vi "Car Wash Client.vi"() -> ()   [LabVIEW 2024]
uses:
  Control 1.ctl
  Global Varibles.vi
  <vilib>/Utility/file.llb/Write Delimited Spreadsheet (string).vi
panel:
  out "error out":errorcluster
  in  "Main Tab":T1(tab)
  in  "Register Button":bool
  in  "Login Button":bool
  in  "Login Back Button":bool
  in  "Login Password":string
  in  "Login Username":string
  out "Login LED":bool
  in  "Login User Button":bool
  in  "Register Username":string
  in  "Register Password":string
  in  "Register Back Button":bool
  in  "Register User Button":bool
  in  "Economy Wash Button":bool
  in  "Deluxe Wash Button":bool
  out "Elapsed Time":dbl
  out "Car Wash Main Tab":enum32{"Deluxe 1"}(tab)
  in  "Stop Button":bool
  out "Vehicle Out of Position":bool
  in  "Car Wash Indicators":enum32{"Page 1"}(tab)
  out "Under Body Wash":bool
  out "Soap Application":bool
  out "Main High Pressure Wash":bool
  out "Clear Water Rinse":bool
  out "Air Dry":bool
  out "Car Wash Simulation Switches":enum32{"Page 1", "Page 2"}(tab)
  in  "Air Dry Position Switch":bool
  in  "Main Wash Position Switch":bool
  in  "Underbody Wash Position Switch":bool
  out "Remaining Time":dbl
  # "Automated Car Wash"
  # "Choose Wash Type"
  # "Deluxe Wash"
  # "Economy Wash"
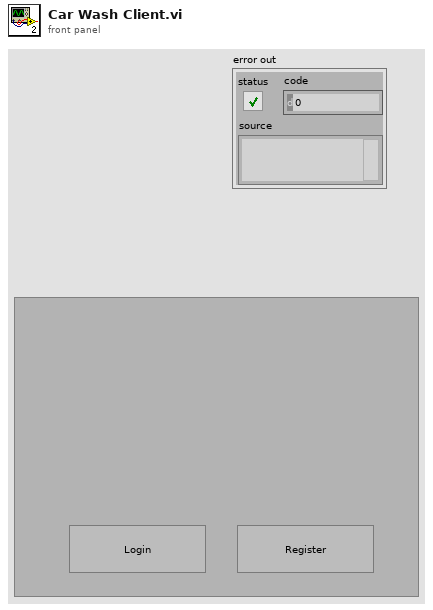
[diagram p1: front panel]
types:
  T1 = enum32{"Login or Register Page", "Login Page", "Register Page", "Choose Car Wash"}
  T2 = typedef "Control 1.ctl" = enum16{"Init", "Wait", "Button Selection", "Login or Register", "Underbody Wash", "Main Wash", "Air Dry", "Log Data"}
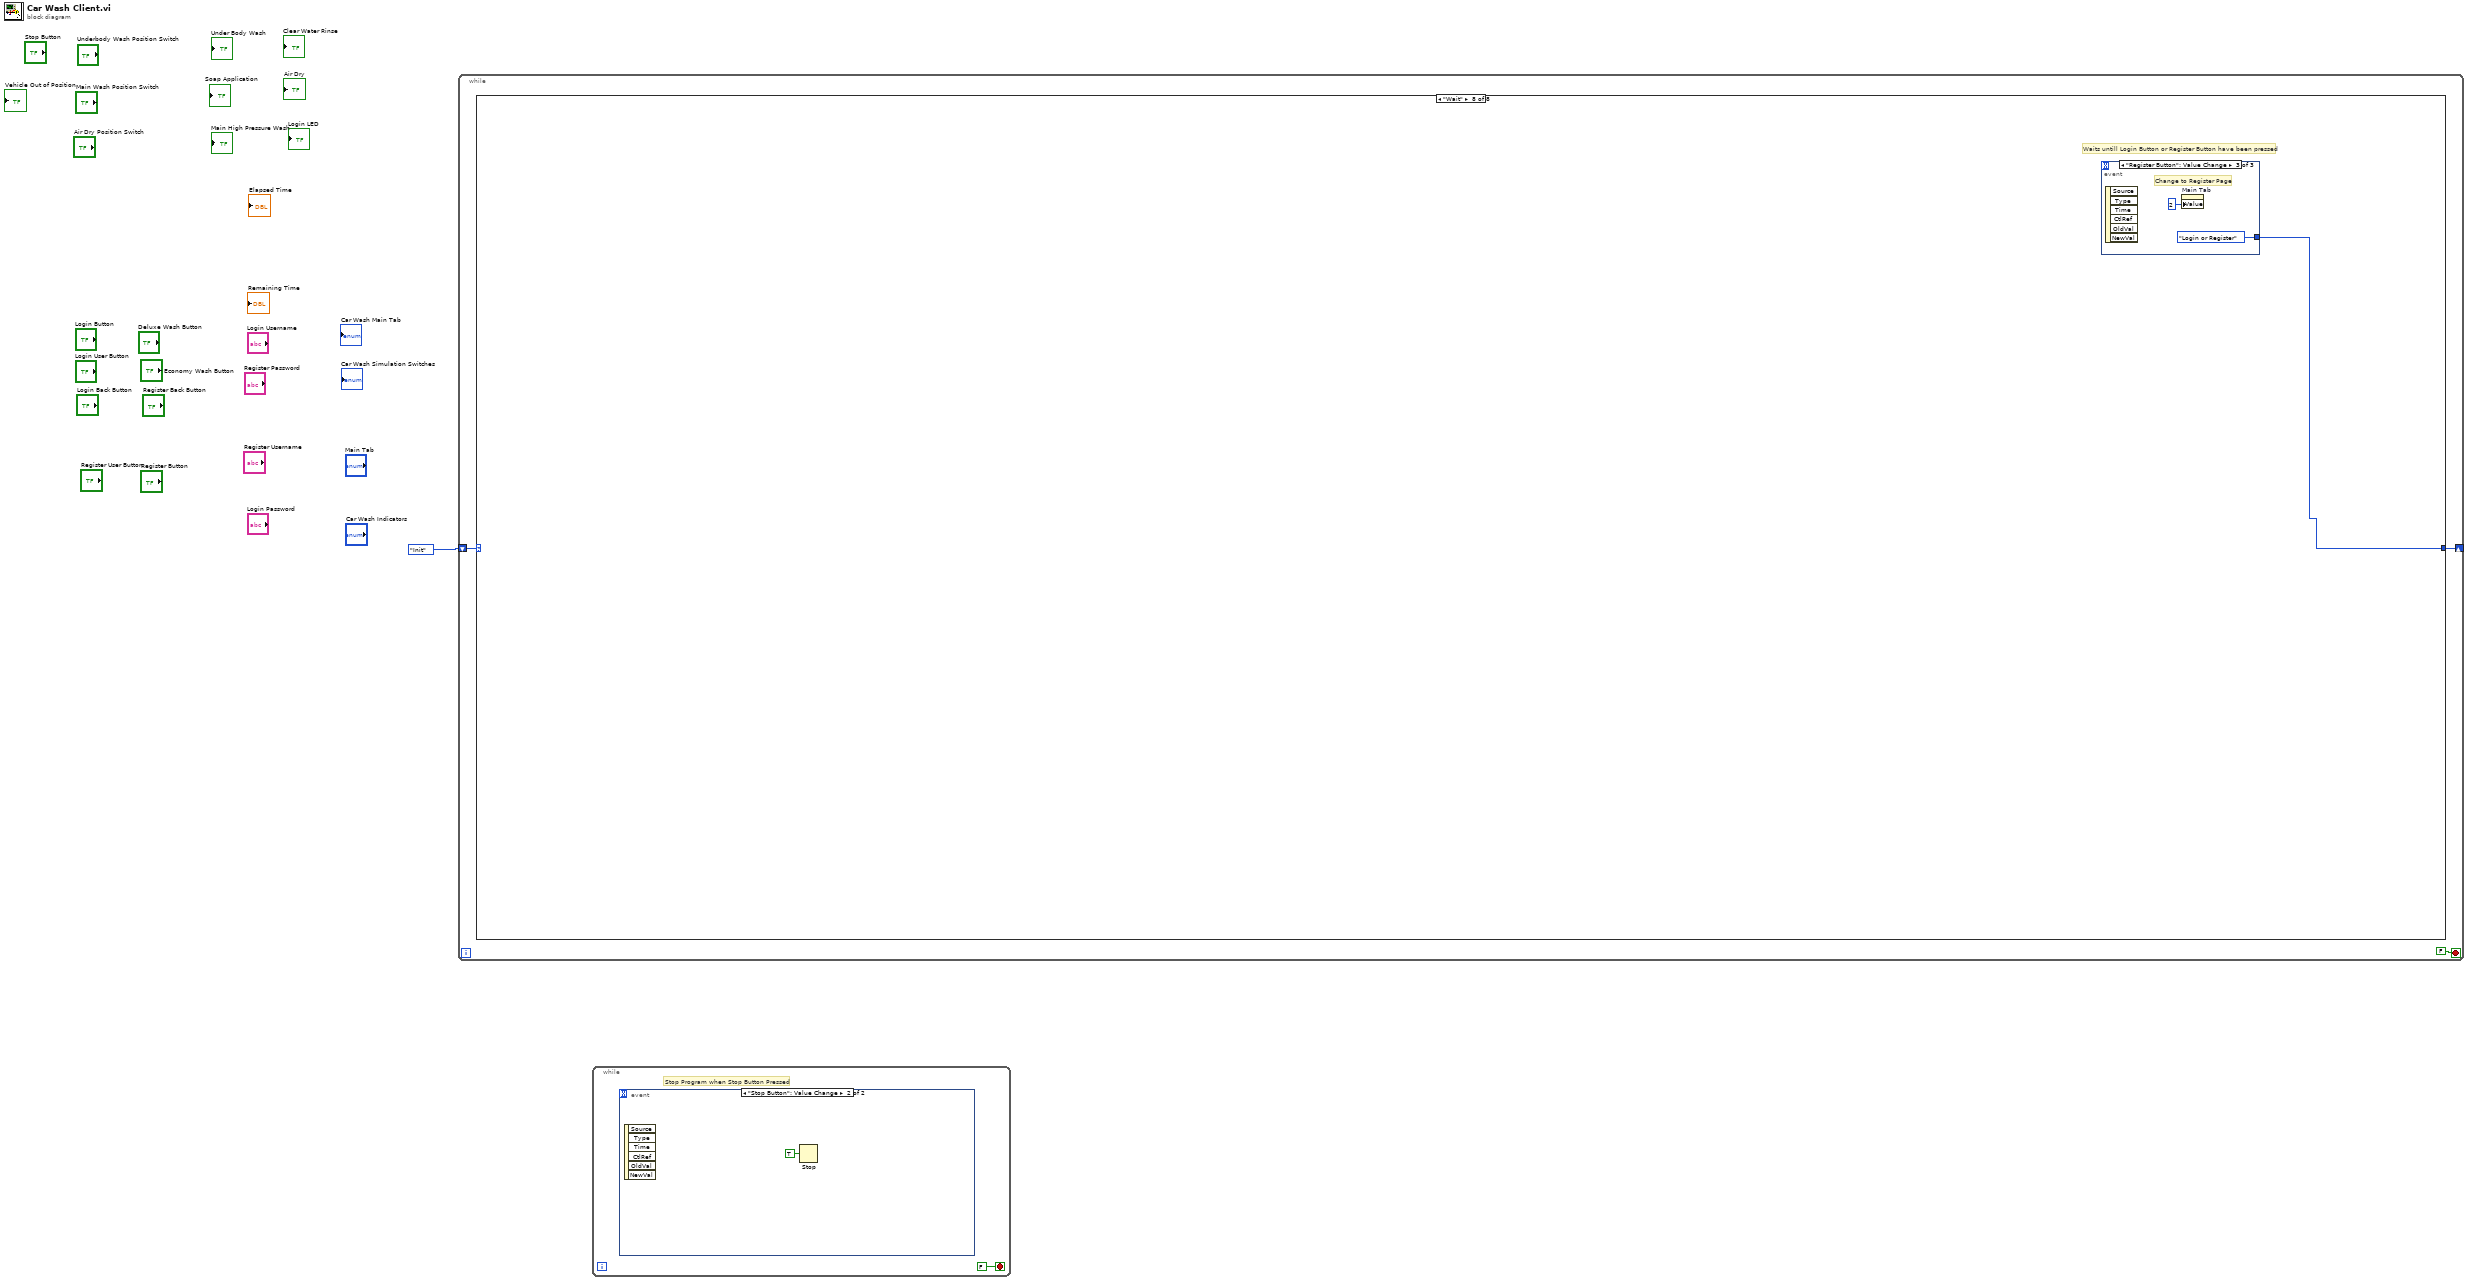
[diagram p0: block diagram]
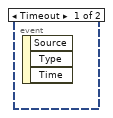
[diagram p2: hidden frame]
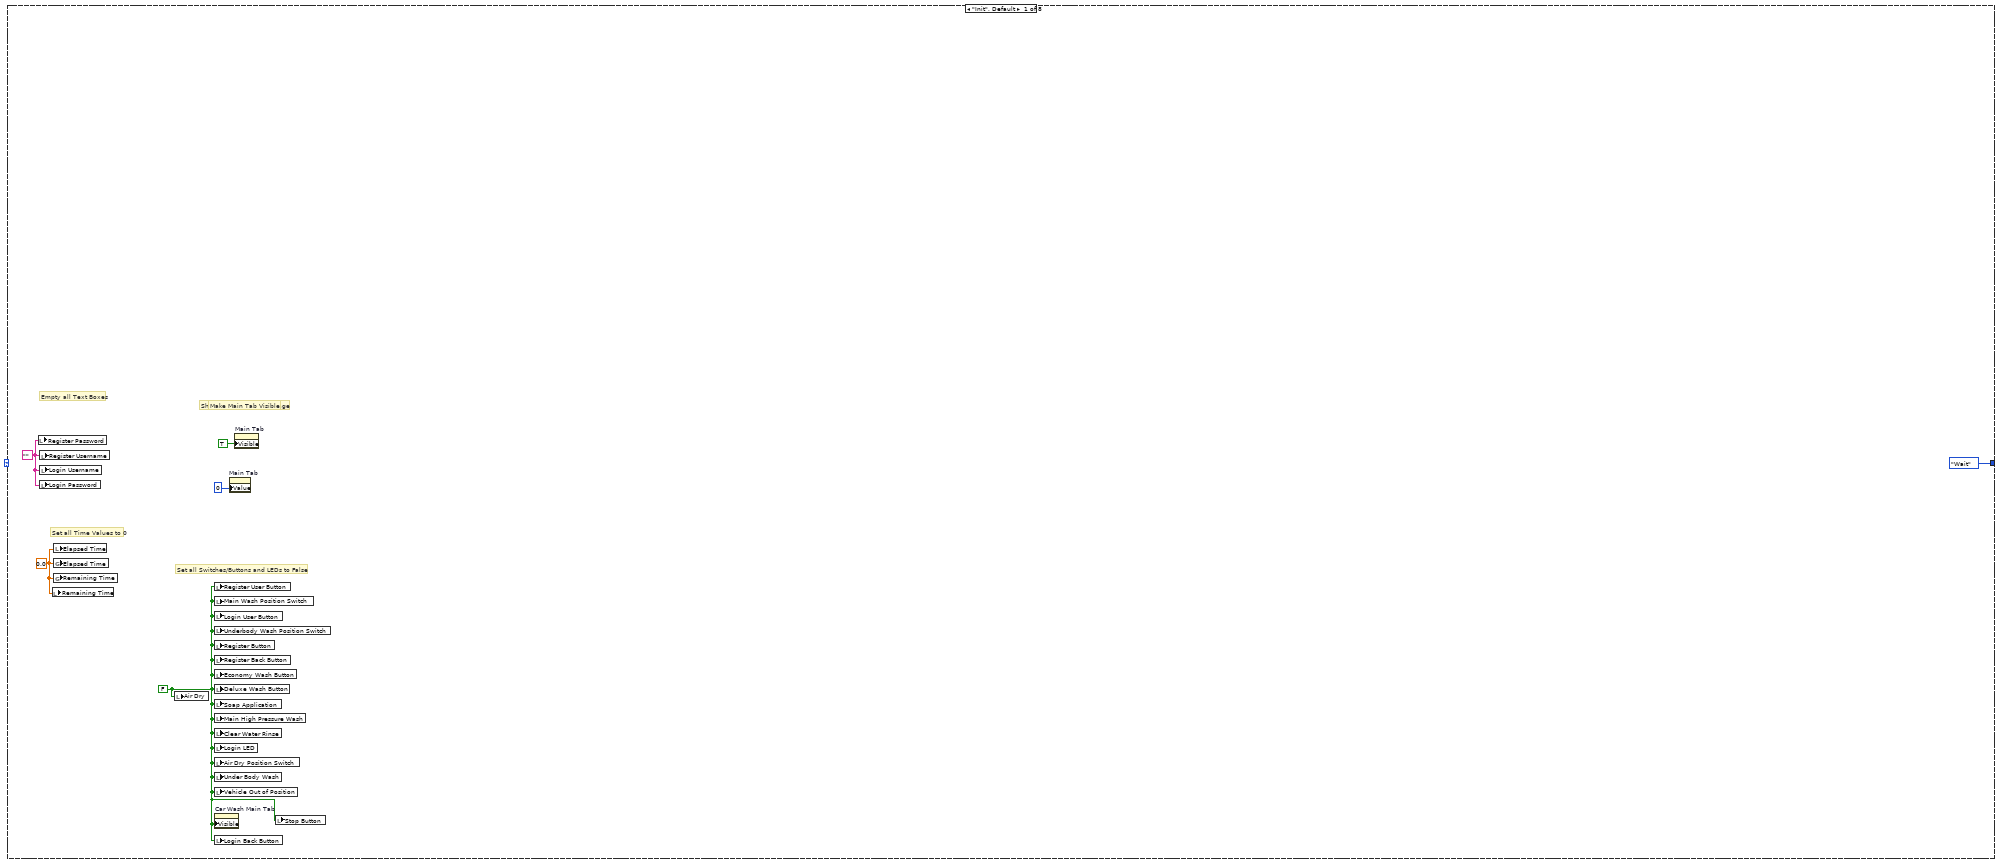
[diagram p3: hidden frame]
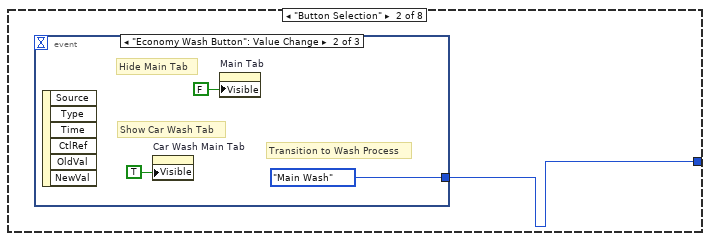
[diagram p4: hidden frame]
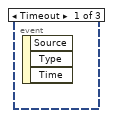
[diagram p5: hidden frame]
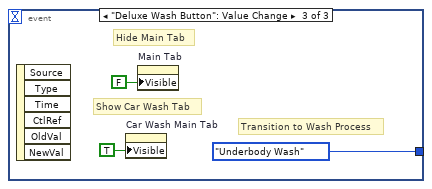
[diagram p6: hidden frame]
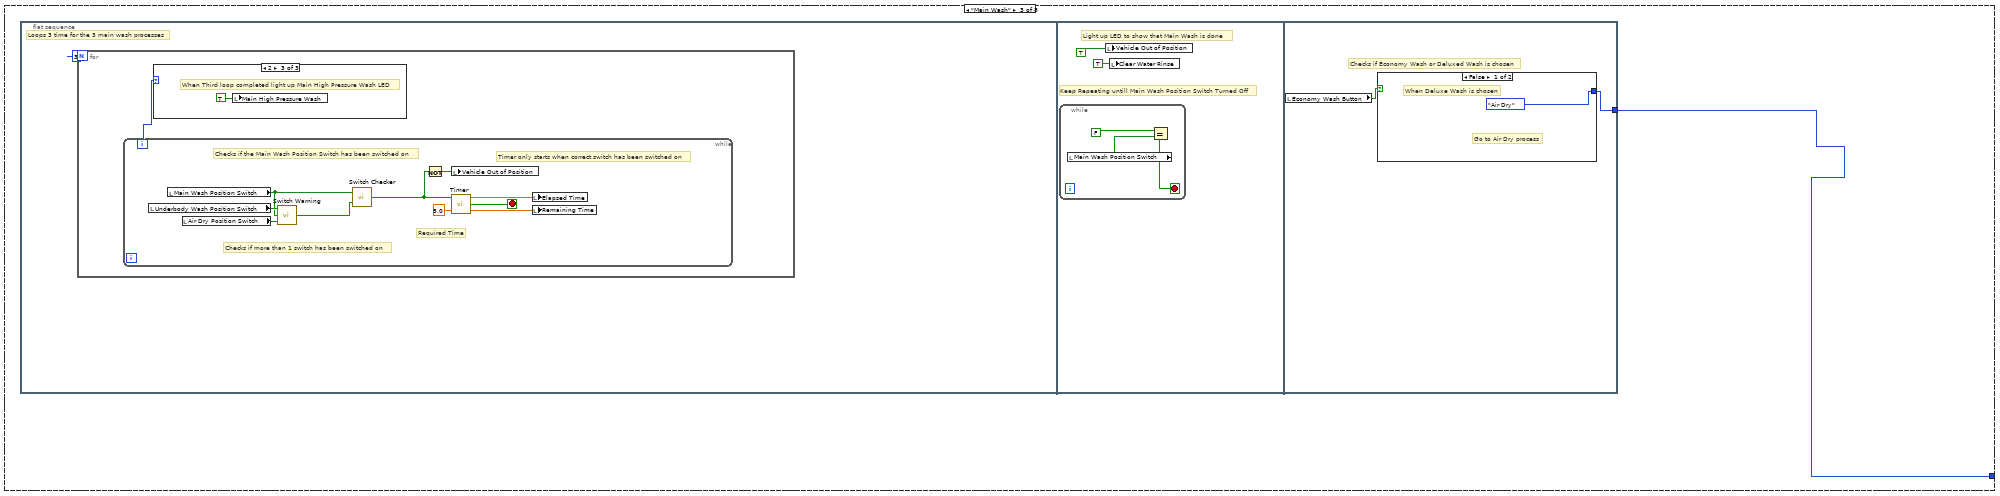
[diagram p7: hidden frame]
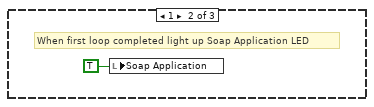
[diagram p9: hidden frame]
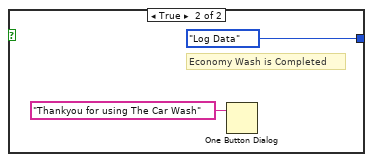
[diagram p10: hidden frame]
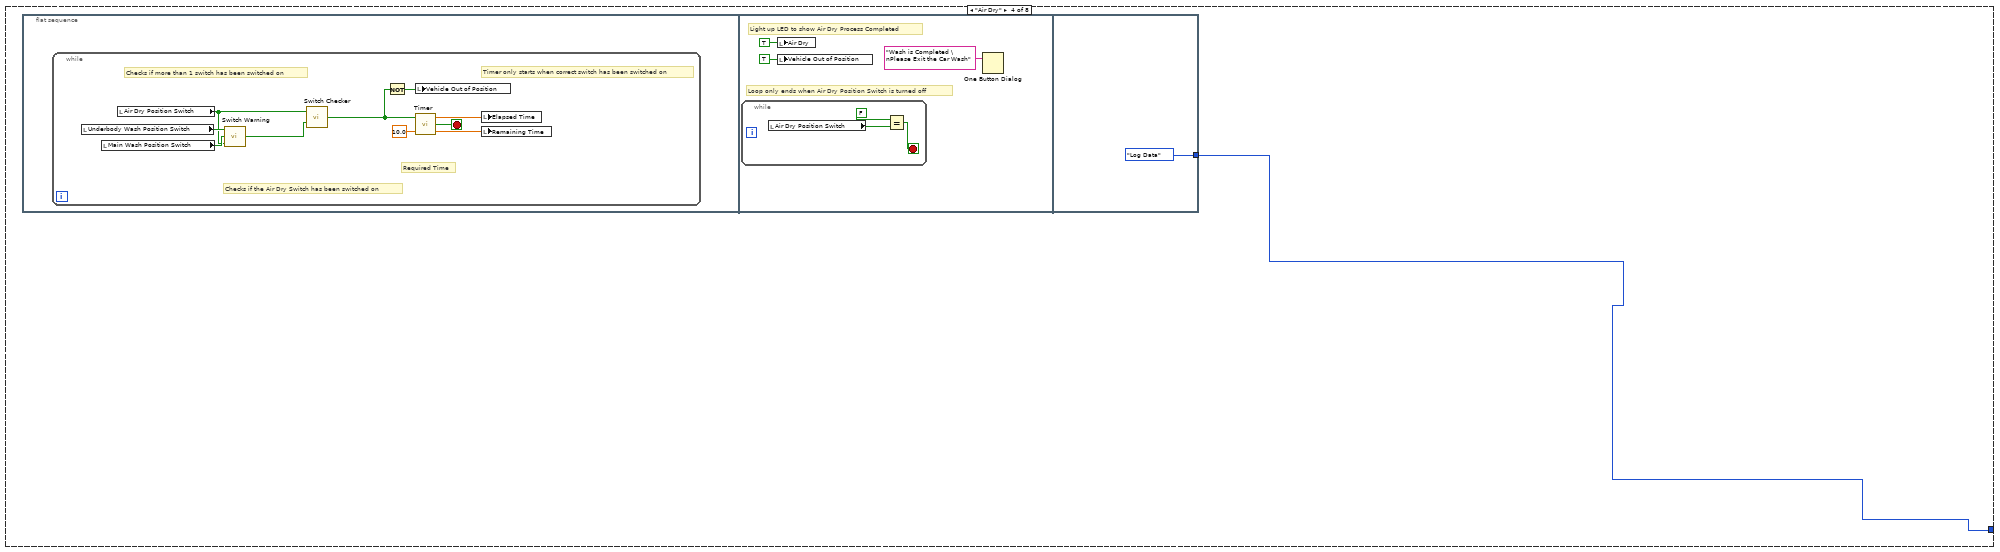
[diagram p11: hidden frame]
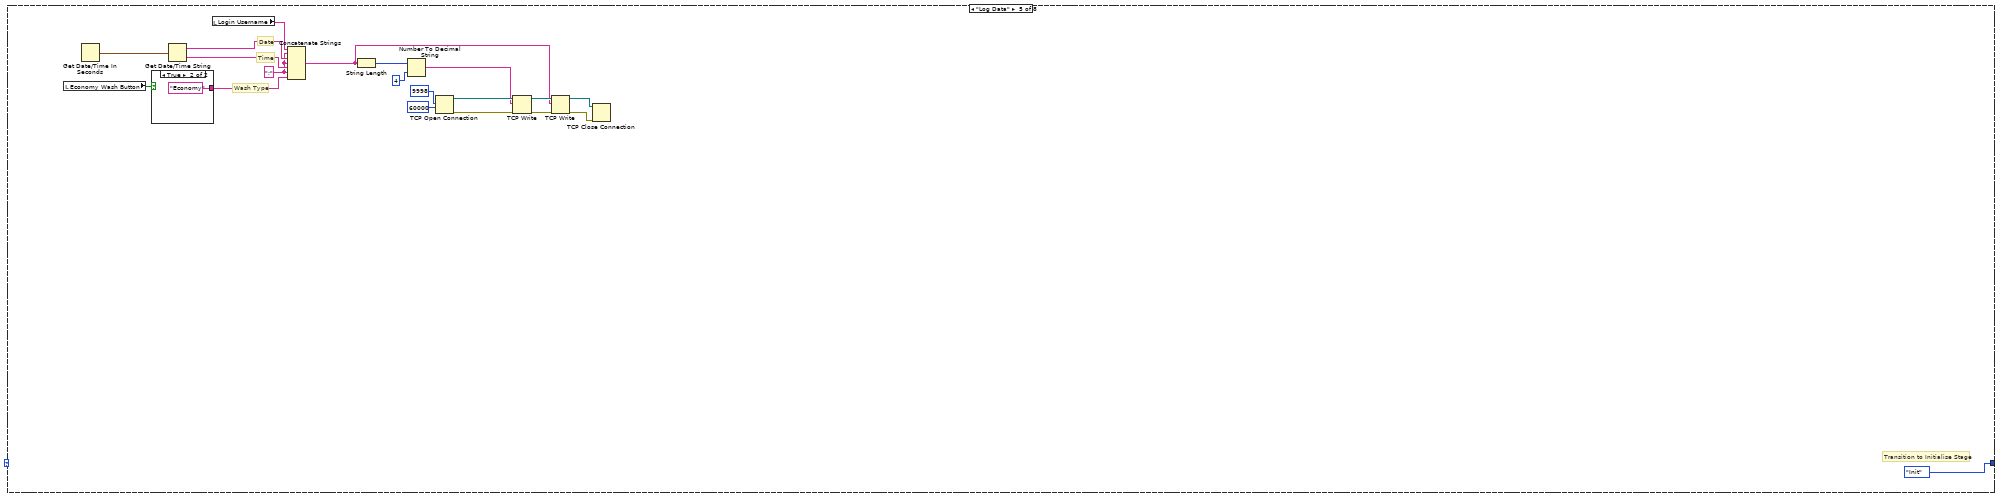
[diagram p12: hidden frame]
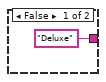
[diagram p13: hidden frame]
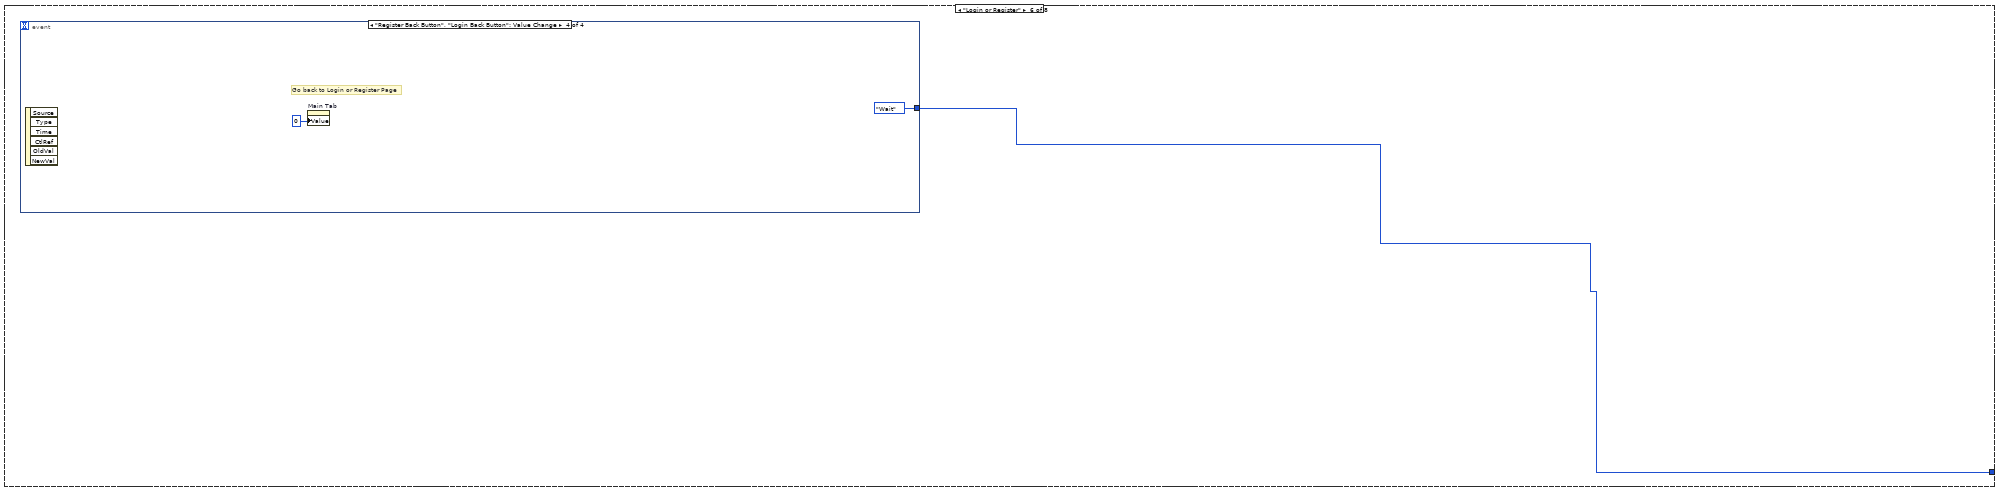
[diagram p14: hidden frame]
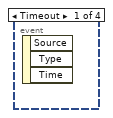
[diagram p15: hidden frame]
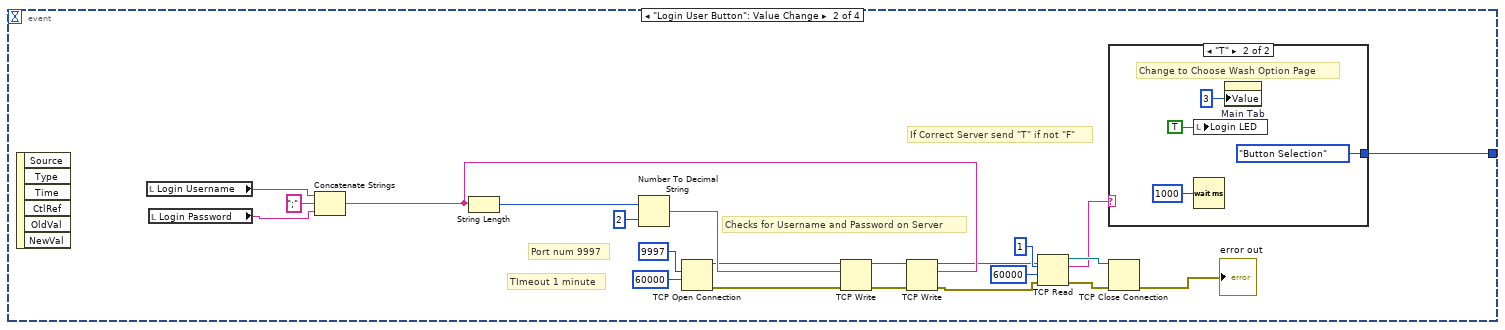
[diagram p16: hidden frame]
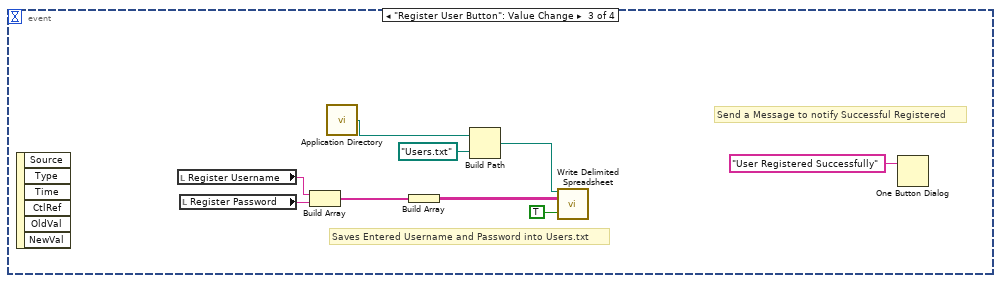
[diagram p18: hidden frame]
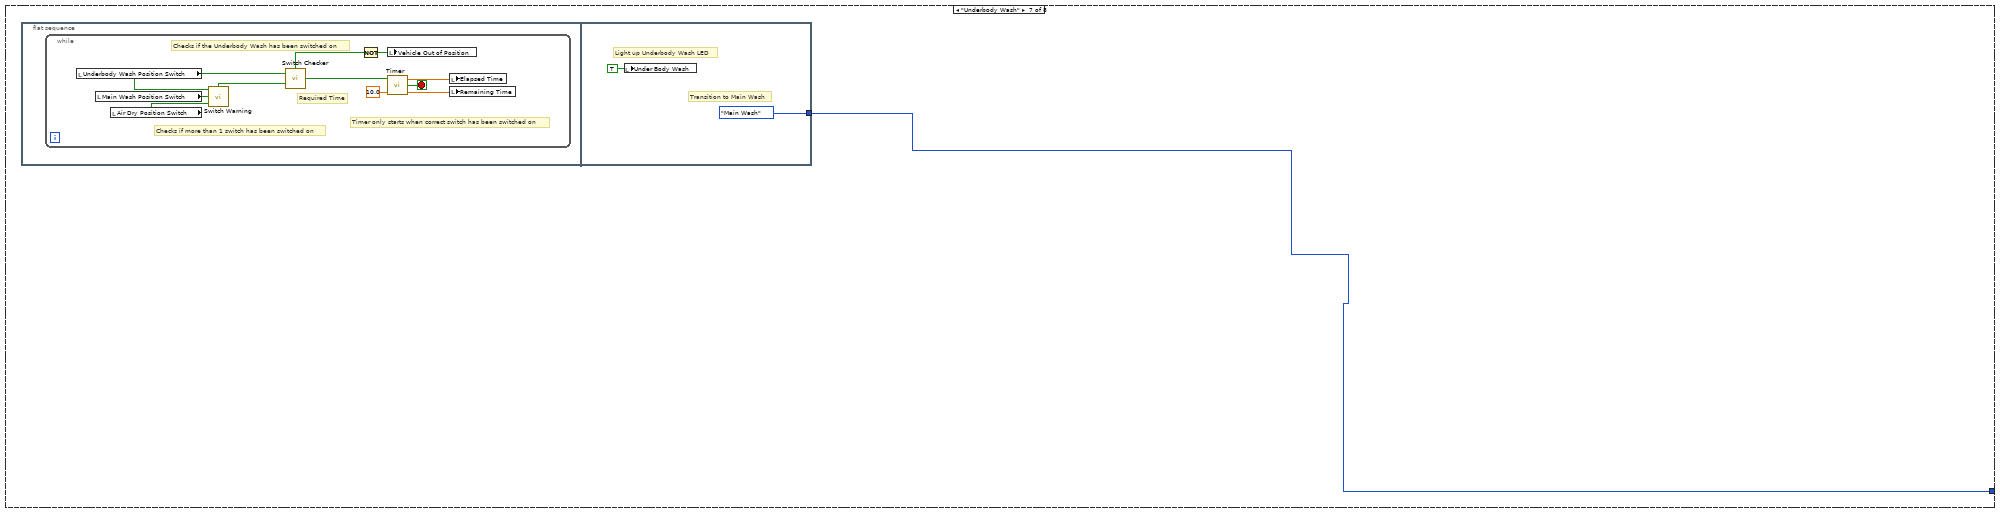
[diagram p19: hidden frame]
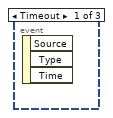
[diagram p20: hidden frame]
diagram:
  n1 = while {
    shift-right: [w3] -> _
    shift-left: Control_1."Init" -> [w4]
    stop <- FALSE stop-if-true
    n2 = case shown="\"Wait\"" w4 {
      tunnel: [Control_1."Wait" w11 w18 w43 Control_1."Init" w83 w121 w134] -> w3
      frame "Init", Default {
        w6 = ""
        w9 = 0.0 ("Elapsed Time")
        w5 = FALSE
        # "Show Login or Register Page"
        # "Make Main Tab Visible"
        # "Empty all Text Boxes"
        # "Set all Time Values to 0"
        # "Set all Switches/Buttons and LEDs to False"
        n3 = local write "Register Password"(w6) -> ()
        n4 = local write "Register Username"(w6) -> ()
        n5 = local write "Login Username"(w6) -> ()
        n6 = local write "Login Password"(w6) -> ()
        n7 = local write "Remaining Time"(w9) -> ()
        n8 = local write "Elapsed Time"(w9) -> ()
        n9 = global write "Global Varibles.vi" "Elapsed Time"(w9) -> ()
        n10 = global write "Global Varibles.vi" "Remaining Time"(w9) -> ()
        n11 = local write "Air Dry"(w5) -> ()
        n12 = local write "Register User Button"(w5) -> ()
        n13 = local write "Main Wash Position Switch"(w5) -> ()
        n14 = local write "Login User Button"(w5) -> ()
        n15 = local write "Underbody Wash Position Switch"(w5) -> ()
        n16 = local write "Register Button"(w5) -> ()
        n17 = local write "Register Back Button"(w5) -> ()
        n18 = local write "Economy Wash Button"(w5) -> ()
        n19 = local write "Deluxe Wash Button"(w5) -> ()
        n20 = local write "Soap Application"(w5) -> ()
        n21 = local write "Main High Pressure Wash"(w5) -> ()
        n22 = local write "Clear Water Rinse"(w5) -> ()
        n23 = local write "Login LED"(w5) -> ()
        n24 = local write "Air Dry Position Switch"(w5) -> ()
        n25 = local write "Under Body Wash"(w5) -> ()
        n26 = local write "Vehicle Out of Position"(w5) -> ()
        n27 = property on="Car Wash Main Tab" class="TabCtl (strict)"("Visible"=w5) -> ()  [unwired: 2 in, 2 out]
        n28 = local write "Login Back Button"(w5) -> ()
        n29 = property on="Main Tab" class="TabCtl (strict)"("Value"=0) -> ()  [unwired: 2 in, 2 out]
        n30 = property on="Main Tab" class="TabCtl (strict)"("Visible"=TRUE) -> ()  [unwired: 2 in, 2 out]
        n31 = local write "Stop Button"(w5) -> ()
      }
      frame "Button Selection" {
        n32 = event shown="[1] \"Economy Wash Button\": Value Change" {
          selector: _ -> [_ _ _]
          dyn-events: _ -> [_ _ _]
          timeout: _ -> [_ _ _]
          tunnel: [_ Control_1."Main Wash" Control_1."Underbody Wash"] -> w11
          event Timeout {
            n33 = event-data() -> ()  [unwired: 1 in, 3 out]
          }
          event "Economy Wash Button": Value Change {
            # "Transition to Wash Process"
            # "Show Car Wash Tab"
            # "Hide Main Tab"
            n34 = event-data() -> ()  [unwired: 1 in, 6 out]
            n35 = property on="Car Wash Main Tab" class="TabCtl (strict)"("Visible"=TRUE) -> ()  [unwired: 2 in, 2 out]
            n36 = property on="Main Tab" class="TabCtl (strict)"("Visible"=FALSE) -> ()  [unwired: 2 in, 2 out]
          }
          event "Deluxe Wash Button": Value Change {
            # "Transition to Wash Process"
            # "Hide Main Tab"
            # "Show Car Wash Tab"
            n37 = event-data() -> ()  [unwired: 1 in, 6 out]
            n38 = property on="Car Wash Main Tab" class="TabCtl (strict)"("Visible"=TRUE) -> ()  [unwired: 2 in, 2 out]
            n39 = property on="Main Tab" class="TabCtl (strict)"("Visible"=FALSE) -> ()  [unwired: 2 in, 2 out]
          }
        }
      }
      frame "Main Wash" {
        n40 = flat-sequence {
          tunnel: [w38] -> w18
          frame #0 {
            # "Loops 3 time for the 3 main wash processes"
            n41 = for {
              N: 3 -> [_]
              i -> [w20]
              n42 = while {
                stop <- w23 stop-if-true
                # "Timer only starts when correct switch has been switched on"
                # "Required Time"
                # "Checks if the Main Wash Position Switch has been switched on"
                # "Checks if more than 1 switch has been switched on"
                n43 = local read "Underbody Wash Position Switch"() -> (w30:bool)
                n44 = local read "Main Wash Position Switch"() -> (w24:bool)
                n45 = local read "Air Dry Position Switch"() -> (w32:bool)
                n46 = call "Switch Warning.vi"("Air Dry Switch"=w32, "Main Wash Switch"=w24, "Underbody Switch A"=w30) -> ("Switch Warning"=w31:bool)
                n47 = call "Switch Checker.vi"("Warning"=w31, "Correct Switch"=w24) -> (0:w28:bool)
                n48 = Not(x=w28) -> (.not. x?=w29:bool)
                n49 = local write "Vehicle Out of Position"(w29) -> ()
                n50 = call "Timer.vi"("Set Timer"=5.0, "Start"=w28) -> ("Remaining Time"=w26:dbl, "End Loop"=w23:bool, "Elapsed Time"=w25:dbl)  [unwired: 1 in]
                n51 = local write "Elapsed Time"(w25) -> ()
                n52 = local write "Remaining Time"(w26) -> ()
              }
              n53 = case shown="2" w20 {
                frame 0, Default {
                }
                frame 1 {
                  # "When first loop completed light up Soap Application LED"
                  n54 = local write "Soap Application"(TRUE ("Soap Application")) -> ()
                }
                frame 2 {
                  # "When Third loop completed light up Main High Pressure Wash LED"
                  n55 = local write "Main High Pressure Wash"(TRUE ("Main High Pressure Wash")) -> ()
                }
              }
            }
          }
          frame #1 {
            # "Light up LED to show that Main Wash is done"
            # "Keep Repeating untill Main Wash Position Switch Turned Off"
            n56 = while {
              stop <- w35 stop-if-true
              n57 = local read "Main Wash Position Switch"() -> (w36:bool)
              n58 = Equal?(x=FALSE, y=w36) -> (x = y?=w35:bool)
            }
            n59 = local write "Vehicle Out of Position"(TRUE) -> ()
            n60 = local write "Clear Water Rinse"(TRUE ("Clear Water Rinse")) -> ()
          }
          frame #2 {
            # "Checks if Economy Wash or Deluxed Wash is chosen"
            n61 = local read "Economy Wash Button"() -> (w39:bool)
            n62 = case shown="False" w39 {
              tunnel: [Control_1."Air Dry" Control_1."Log Data"] -> w38
              frame False {
                # "Go to Air Dry process"
                # "When Deluxe Wash is chosen"
              }
              frame True {
                # "Economy Wash is Completed"
                n63 = One Button Dialog(message="Thankyou for using The Car Wash") -> ()  [unwired: 1 in, 1 out]
              }
            }
          }
        }
      }
      frame "Air Dry" {
        n64 = flat-sequence {
          tunnel: [Control_1."Log Data"] -> w43
          frame #0 {
            n65 = while {
              stop <- w49 stop-if-true
              # "Timer only starts when correct switch has been switched on"
              # "Required Time"
              # "Checks if the Air Dry Switch has been switched on"
              # "Checks if more than 1 switch has been switched on"
              n66 = local read "Underbody Wash Position Switch"() -> (w52:bool)
              n67 = local read "Main Wash Position Switch"() -> (w45:bool)
              n68 = local read "Air Dry Position Switch"() -> (w44:bool)
              n69 = call "Switch Warning.vi"("Air Dry Switch"=w44, "Main Wash Switch"=w45, "Underbody Switch A"=w52) -> ("Switch Warning"=w53:bool)
              n70 = call "Switch Checker.vi"("Warning"=w53, "Correct Switch"=w44) -> (0:w50:bool)
              n71 = Not(x=w50) -> (.not. x?=w51:bool)
              n72 = local write "Vehicle Out of Position"(w51) -> ()
              n73 = call "Timer.vi"("Set Timer"=10.0, "Start"=w50) -> ("Remaining Time"=w47:dbl, "End Loop"=w49:bool, "Elapsed Time"=w46:dbl)  [unwired: 1 in]
              n74 = local write "Elapsed Time"(w46) -> ()
              n75 = local write "Remaining Time"(w47) -> ()
            }
          }
          frame #1 {
            # "Loop only ends when Air Dry Position Switch is turned off"
            # "Light up LED to show Air Dry Process Completed"
            n76 = while {
              stop <- w57 stop-if-true
              n77 = local read "Air Dry Position Switch"() -> (w59:bool)
              n78 = Equal?(x=FALSE, y=w59) -> (x = y?=w57:bool)
            }
            n79 = local write "Air Dry"(TRUE ("Air Dry")) -> ()
            n80 = local write "Vehicle Out of Position"(TRUE) -> ()
            n81 = One Button Dialog(message="Wash is Completed \nPlease Exit the Car Wash") -> ()  [unwired: 1 in, 1 out]
          }
          frame #2 {
          }
        }
      }
      frame "Log Data" {
        w74 = ";"
        # "Transition to Initialise Stage"
        # "Wash Type"
        # "Time"
        # "Date"
        n82 = local read "Economy Wash Button"() -> (w76:bool)
        n83 = Get Date/Time In Seconds() -> (seconds since 1Jan1904=w80:timestamp)
        n84 = case shown="True" w76 {
          tunnel: ["Deluxe" "Economy"] -> w75
          frame False {
          }
          frame True {
          }
        }
        n85 = Get Date/Time String(seconds (now)=w80) -> (date string=w78:string, time string=w77:string)  [unwired: 2 in]
        n86 = local read "Login Username"() -> (w79:string)
        n87 = Concatenate Strings "Concatenate Strings"(w79, w74, w78, w74, w77, w74, w75) -> (w62:string)
        n88 = String Length(string=w62) -> (length=w65:i32)
        n89 = Number To Decimal String(number=w65, width (-)=i16 4) -> (decimal integer string=w63:string)
        n90 = TCP Open Connection(remote port or service name=u16 9998, timeout ms (60000)=60000) -> (connection ID=w71:refnum<k5>, error out=w68:errorcluster)  [unwired: 3 in]
        n91 = TCP Write(connection ID=w71, data in=w63, error in (no error)=w68) -> (connection ID out=w70:refnum<k5>, error out=w67:errorcluster)  [unwired: 1 in, 1 out]
        n92 = TCP Write(connection ID=w70, data in=w62, error in (no error)=w67) -> (connection ID out=w69:refnum<k5>, error out=w66:errorcluster)  [unwired: 1 in, 1 out]
        n93 = TCP Close Connection(connection ID=w69, error in (no error)=w66) -> ()  [unwired: 1 in, 2 out]
      }
      frame "Login or Register" {
        n94 = event shown="[3] \"Register Back Button\", \"Login Back Button\": Value Change" {
          selector: _ -> [_ _ _ _]
          dyn-events: _ -> [_ _ _ _]
          timeout: _ -> [_ _ _ _]
          tunnel: [_ w85 _ Control_1."Wait"] -> w83
          event Timeout {
            n95 = event-data() -> ()  [unwired: 1 in, 3 out]
          }
          event "Login User Button": Value Change {
            # "If Correct Server send \"T\" if not \"F\""
            # "Checks for Username and Password on Server"
            # "TImeout 1 minute"
            # "Port num 9997"
            n96 = event-data() -> ()  [unwired: 1 in, 6 out]
            n97 = local read "Login Username"() -> (w89:string)
            n98 = local read "Login Password"() -> (w88:string)
            n99 = Concatenate Strings "Concatenate Strings"(w89, ";" ("string"), w88) -> (w96:string)
            n100 = String Length(string=w96) -> (length=w90:i32)
            n101 = Number To Decimal String(number=w90, width (-)=i16 2) -> (decimal integer string=w95:string)
            n102 = TCP Open Connection(remote port or service name=u16 9997, timeout ms (60000)=60000) -> (connection ID=w91:refnum<k5>, error out=w97:errorcluster)  [unwired: 3 in]
            n103 = TCP Write(connection ID=w91, data in=w95, error in (no error)=w97) -> (connection ID out=w92:refnum<k5>, error out=w98:errorcluster)  [unwired: 1 in, 1 out]
            n104 = TCP Write(connection ID=w92, data in=w96, error in (no error)=w98) -> (connection ID out=w93:refnum<k5>, error out=w99:errorcluster)  [unwired: 1 in, 1 out]
            n105 = TCP Read(connection ID=w93, bytes to read=1, error in (no error)=w99, 9:60000 ("timeout ms (25000)")) -> (connection ID out=w94:refnum<k5>, data out=w86:string, error out=w100:errorcluster)  [unwired: 1 in]
            n106 = case shown="\"T\"" w86 {
              tunnel: [_ Control_1."Button Selection"] -> w85
              frame "F", Default {
              }
              frame "T" {
                # "Change to Choose Wash Option Page"
                n107 = local write "Login LED"(TRUE ("Login LED")) -> ()
                n108 = Wait (ms)(milliseconds to wait=u32 1000) -> ()  [unwired: 1 out]
                n109 = property on="Main Tab" class="TabCtl (strict)"("Value"=3) -> ()  [unwired: 2 in, 2 out]
              }
            }
            n110 = TCP Close Connection(connection ID=w94, error in (no error)=w100) -> (error out=→"error out":errorcluster)  [unwired: 1 in, 1 out]
          }
          event "Register User Button": Value Change {
            # "Send a Message to notify Successful Registered"
            # "Saves Entered Username and Password into Users.txt"
            n111 = event-data() -> ()  [unwired: 1 in, 6 out]
            n112 = local read "Register Username"() -> (w114:string)
            n113 = local read "Register Password"() -> (w113:string)
            n114 = Build Array "Build Array"(w114, w113) -> (w112:string[])
            n115 = call <vilib>:"Application Directory.vi"() -> ("Application Directory"=w115:path)
            n116 = Build Array "Build Array"(w112) -> (w111:string[][])
            n117 = Build Path(base path=w115, name or relative path=path "Users.txt") -> (appended path=w116:path)
            n118 = call-poly <vilib>:"Write Delimited Spreadsheet.vi"("file path (dialog if empty)"=w116, "2D data"=w111, "append to file? (new file:F)"=TRUE) -> ()  [unwired: 11 in, 2 out]
            n119 = One Button Dialog(message="User Registered Successfully") -> ()  [unwired: 1 in, 1 out]
          }
          event "Register Back Button", "Login Back Button": Value Change {
            # "Go back to Login or Register Page"
            n120 = event-data() -> ()  [unwired: 1 in, 6 out]
            n121 = property on="Main Tab" class="TabCtl (strict)"("Value"=0) -> ()  [unwired: 2 in, 2 out]
          }
        }
      }
      frame "Underbody Wash" {
        n122 = flat-sequence {
          tunnel: [Control_1."Main Wash"] -> w121
          frame #0 {
            n123 = while {
              stop <- w126 stop-if-true
              # "Timer only starts when correct switch has been switched on"
              # "Required Time"
              # "Checks if the Underbody Wash has been switched on"
              # "Checks if more than 1 switch has been switched on"
              n124 = local read "Underbody Wash Position Switch"() -> (w129:bool)
              n125 = local read "Main Wash Position Switch"() -> (w131:bool)
              n126 = local read "Air Dry Position Switch"() -> (w130:bool)
              n127 = call "Switch Warning.vi"("Air Dry Switch"=w130, "Main Wash Switch"=w131, "Underbody Switch A"=w129) -> ("Switch Warning"=w122:bool)
              n128 = call "Switch Checker.vi"("Warning"=w122, "Correct Switch"=w129) -> (0:w127:bool)
              n129 = Not(x=w127) -> (.not. x?=w128:bool)
              n130 = local write "Vehicle Out of Position"(w128) -> ()
              n131 = call "Timer.vi"("Set Timer"=10.0, "Start"=w127) -> ("Remaining Time"=w124:dbl, "End Loop"=w126:bool, "Elapsed Time"=w123:dbl)  [unwired: 1 in]
              n132 = local write "Elapsed Time"(w123) -> ()
              n133 = local write "Remaining Time"(w124) -> ()
            }
          }
          frame #1 {
            # "Transition to Main Wash"
            # "Light up Underbody Wash LED"
            n134 = local write "Under Body Wash"(TRUE) -> ()
          }
        }
      }
      frame "Wait" {
        # "Waits untill Login Button or Register Button have been pressed"
        n135 = event shown="[2] \"Register Button\": Value Change" {
          selector: _ -> [_ _ _]
          dyn-events: _ -> [_ _ _]
          timeout: _ -> [_ _ _]
          tunnel: [_ Control_1."Login or Register" Control_1."Login or Register"] -> w134
          event Timeout {
            n136 = event-data() -> ()  [unwired: 1 in, 3 out]
          }
          event "Login Button": Value Change {
            # "Change to Login Page"
            n137 = event-data() -> ()  [unwired: 1 in, 6 out]
            n138 = property on="Main Tab" class="TabCtl (strict)"("Value"=1) -> ()  [unwired: 2 in, 2 out]
          }
          event "Register Button": Value Change {
            # "Change to Register Page"
            n139 = event-data() -> ()  [unwired: 1 in, 6 out]
            n140 = property on="Main Tab" class="TabCtl (strict)"("Value"=2) -> ()  [unwired: 2 in, 2 out]
          }
        }
      }
    }
  }
  n141 = while {
    stop <- FALSE stop-if-true
    # "Stop Program when Stop Button Pressed"
    n142 = event shown="[1] \"Stop Button\": Value Change" {
      selector: _ -> [_ _]
      dyn-events: _ -> [_ _]
      timeout: _ -> [_ _]
      event Timeout {
        n143 = event-data() -> ()  [unwired: 1 in, 3 out]
      }
      event "Stop Button": Value Change {
        n144 = event-data() -> ()  [unwired: 1 in, 6 out]
        n145 = Stop(stop? (T)=TRUE) -> ()
      }
    }
  }
